vi "Simulate Mouse.vi"(7 "SetCursorPos":bool=TRUE, 8 "error in (no error)":errorcluster, 9 "y position":i32=200, 10 "x position":i32=200, 11 "Action":T1(ring)) -> (0 "error out":errorcluster)   [LabVIEW 2017]
doc: "This VI allows you to simulate a mouse action. To perform a click you would need to execute this VI twice, once with mouse down, then with mouse up. You can set the position of the mouse when \"Set mouse position prior to action?\" is true. (0, 0) corresponds to the top left corner of your screen, then the bottom right corner of your screen is your screen resolution e.g. (1920, 1080). \n\nIndividual mouse up and mouse down events allow the simulation of click and hold functionality. For example left mouse down will click and hold left mouse until you simulate mouse up or click the left button of your mouse."
uses:
  User32.dll
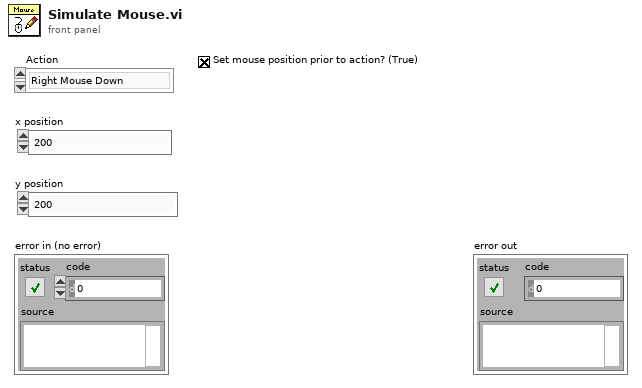
[diagram p1: front panel]
types:
  T1 = enum16{"Right Mouse Down", "Right Mouse Up", "Middle Mouse Down", "Middle Mouse Up", "Left Mouse Down", "Left Mouse Up"}
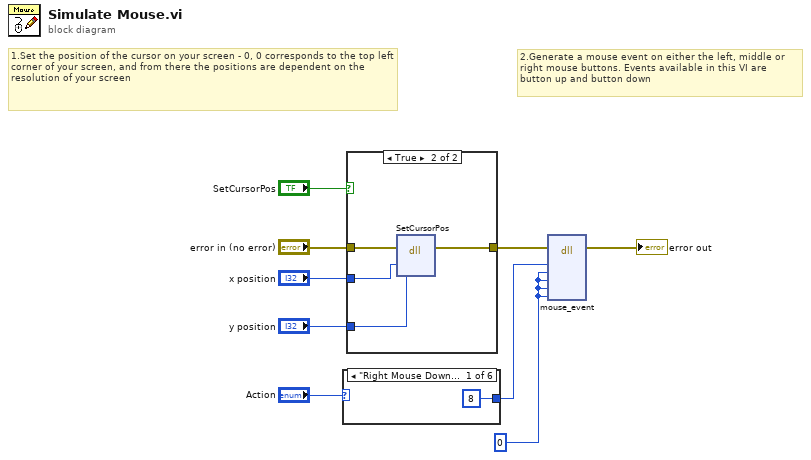
[diagram p0: block diagram]
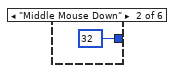
[diagram p3: hidden frame]
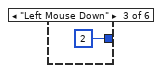
[diagram p4: hidden frame]
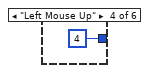
[diagram p5: hidden frame]
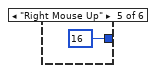
[diagram p6: hidden frame]
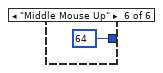
[diagram p7: hidden frame]
diagram:
  w1 = u32 0 ("dwExtraInfo")
  # "1.Set the position of the cursor on your screen - 0, 0 corresponds to the top left corner of your screen, and from there the positions are dependent on the resolution of your screen"
  # "2.Generate a mouse event on either the left, middle or right mouse buttons. Events available in this VI are button up and button down"
  n1 = case shown="\"Right Mouse Down\", Default" "Action" {
    tunnel: [8 32 2 4 16 64] -> w9
    frame "Right Mouse Down", Default {
    }
    frame "Middle Mouse Down" {
    }
    frame "Left Mouse Down" {
    }
    frame "Left Mouse Up" {
    }
    frame "Right Mouse Up" {
    }
    frame "Middle Mouse Up" {
    }
  }
  n2 = case shown="True" "SetCursorPos" {
    tunnel: [w16 w20] -> w6
    tunnel: "error in (no error)" -> [w16 w19]
    tunnel: "x position" -> [_ w18]
    tunnel: "y position" -> [_ w17]
    frame False {
    }
    frame True {
      n3 = dll-call lib="User32.dll" fn="SetCursorPos"(error in=w19, w18, w17) -> (error out=w20:errorcluster)  [unwired: 5 in, 1 out]
    }
  }
  n4 = dll-call lib="user32.dll" fn="mouse_event" label="Mouse_Event"(error in=w6, "dwFlags"=w9, "dx"=w1, "dy"=w1, "dwData"=w1, "dwExtraInfo"=w1) -> (error out=→"error out":errorcluster)  [unwired: 8 in, 1 out]
